vi "poly_loop_timeout_bool.vi"(1 "timeout (2k ms)":i32=2000, 2 "i (reset @ 0)":i32=1) -> (6 "timeout":bool)   [LabVIEW 2015]
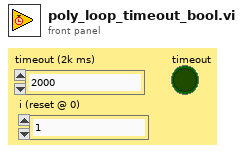
[diagram p1: front panel]
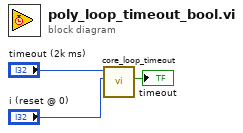
[diagram p0: block diagram]
diagram:
  n1 = call "core_loop_timeout.vi"("i (reset @ 0)"="i (reset @ 0)", "timeout (2k ms)"="timeout (2k ms)") -> ("timeout"=→"timeout":bool)  [unwired: 7 in, 1 out]
